vi "Save Changes.vi"   [LabVIEW 2020, in "nisyscfg.lvlib"]
doc: "Saves changes made to hardware and systems."
uses:
  <vilib>/nisyscfg/nisyscfg.lvlib
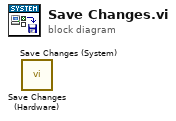
[diagram p0: block diagram]
diagram:
  n1 = call <vilib>:"Save Changes (Hardware).vi"() -> ()  [unwired: 8 in, 4 out]
  n2 = call <vilib>:"Save Changes (System).vi"() -> ()  [unwired: 8 in, 4 out]
